vi "FT_Get_Queue_Status.vi"(0 "Handle":u32) -> (1 "Handle":u32, 2 "FT_Status":u32, 3 "Bytes Waiting":u32)   [LabVIEW 2011]
uses:
  FTD2XX.dll
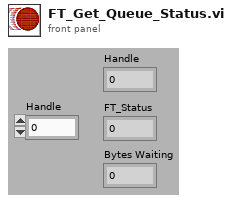
[diagram p1: front panel]
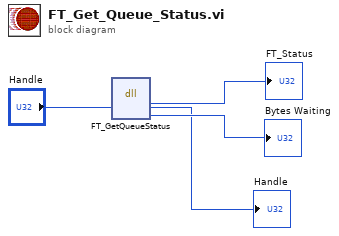
[diagram p0: block diagram]
diagram:
  n1 = dll-call lib="D:/WORK/LabView/#Avesta/D2XX_Functions_7.0/FTD2XX.dll" fn="FT_GetQueueStatus"("Handle"="Handle") -> ("FT_Status"=→"FT_Status":u32, "Handle"=→"Handle":u32, "BytesWaiting"=→"Bytes Waiting":u32)  [unwired: 3 in, 3 out]
